vi "test_hashlib_sha256_hmac.vi"() -> (3 "all_passed":bool)   [LabVIEW 2019]
doc: "Tests HMAC-SHA-256 VIs"
uses:
  <userlib>/_rcpacini/hashlib/hashlib/hashlib.lvlib
panel:
  out "sha256":string[](array[string])
  out "passed":bool[](array[boolean])
  in  "test_cases":T1(array[cluster])
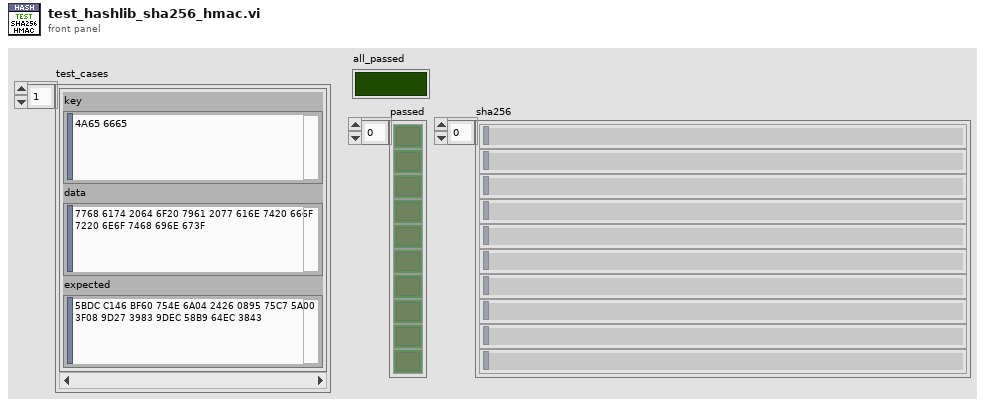
[diagram p1: front panel]
types:
  T1 = cluster{"key":string, "data":string, "expected":string}[]
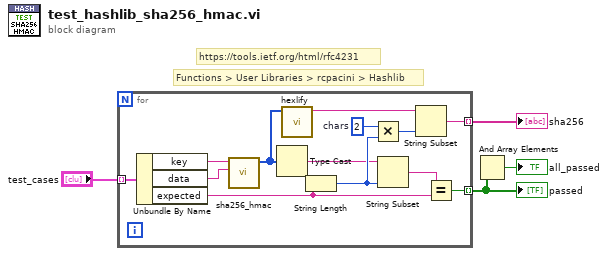
[diagram p0: block diagram]
diagram:
  # "Functions > User Libraries > rcpacini > Hashlib"
  # "https://tools.ietf.org/html/rfc4231"
  n1 = for {
    tunnel: "test_cases" -> [w17] mode=indexing
    tunnel: [w16] -> w3 mode=indexing
    tunnel: [w14] -> w1 mode=indexing
    w11 = 2  # chars
    n2 = Unbundle By Name(w17) -> ("key"=w8:string, "data"=w7:string, "expected"=w15:string)
    n3 = call <userlib>:"sha256_hmac.vi"("data"=w7, "key"=w8) -> ("sha256"=w6:u32[])  [unwired: 9 in]
    n4 = Type Cast(x=w6) -> (*(type *) &x=w10:string)  [unwired: 1 in]
    n5 = call <userlib>:"hexlify.vi"("sha256"=w6) -> ("hex (0-9a-f)"=w5:string)  [unwired: 10 in]
    n6 = String Length(string=w15) -> (length=w13:i32)
    n7 = Multiply(x=w11, y=w13) -> (x*y=w12:i32)
    n8 = String Subset(string=w10, length (rest)=w13) -> (substring=w9:string)  [unwired: 1 in]
    n9 = String Subset(string=w5, length (rest)=w12) -> (substring=w14:string)  [unwired: 1 in]
    n10 = Equal?(x=w9, y=w15) -> (x = y?=w16:bool)
  }
  "passed" <- w3
  "sha256" <- w1
  n11 = And Array Elements(Boolean array=w3) -> (logical AND=→"all_passed":bool)
